vi "Create SBlock (array of pairs).vi"(0 "FPGA Name":string, 5 "Script Path":path, 7 "Common Parameters":T1[](array[typedef]), 9 "Number of repetitions":u16, 11 "error in (no error)":errorcluster) -> (4 "Schedule Block out":refnum<class "Schedule Block.lvclass">, 6 "FPGA Name":string, 15 "error out":errorcluster)   [LabVIEW 2020, in "CIRCUS_uServices.lvlib" / "Run Utilities.lvlib" / "Schedule Block.lvclass"]
uses:
  Schedule Block.lvclass
  Schedule Block.lvclass/Schedule Block.ctl
  TALOS/TALOS_PPL.lvlibp/Interfaces/FPGA Interface/FPGA Interface.lvclass
  TALOS/TALOS_PPL.lvlibp/Support VIs/Global Memory.vi
  TALOS/TALOS_PPL.lvlibp
  Scan SBlock/Parameter name with value - GUI.ctl
  Scan SBlock/Scan SBlock.lvclass
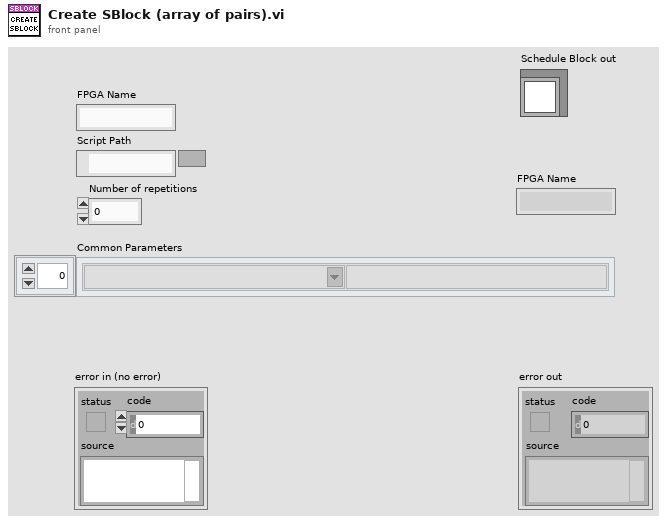
[diagram p1: front panel]
types:
  T1 = typedef "CIRCUS_uServices.lvlib/Run Utilities.lvlib/Scan SBlock.lvclass/Parameter name with value - GUI.ctl" = cluster{"Parameter Name":string, "Parameter Value":string}
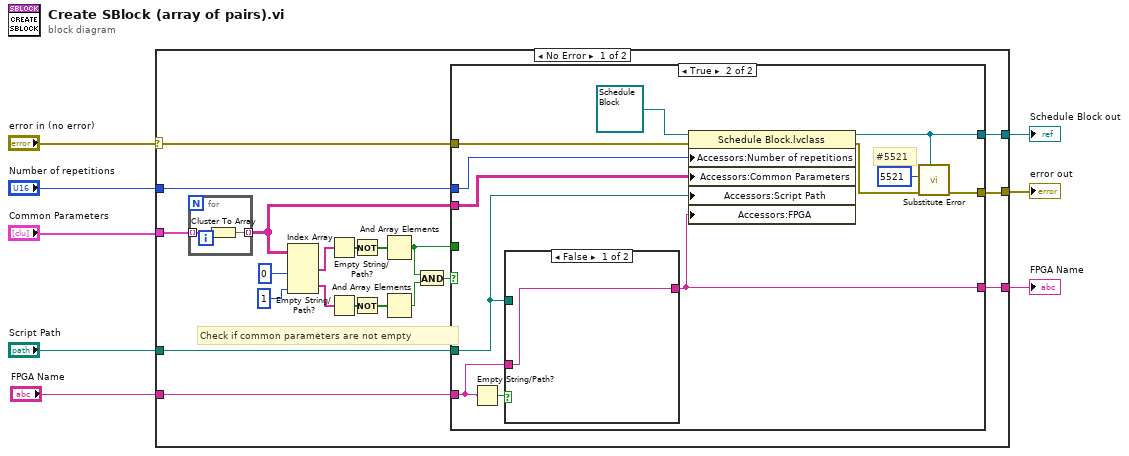
[diagram p0: block diagram]
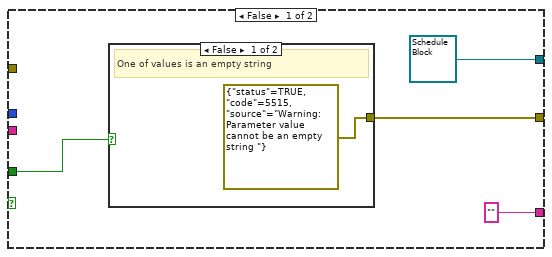
[diagram p2: hidden frame]
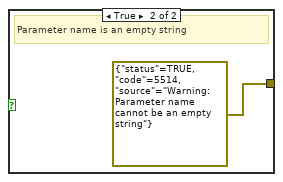
[diagram p3: hidden frame]
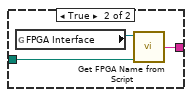
[diagram p4: hidden frame]
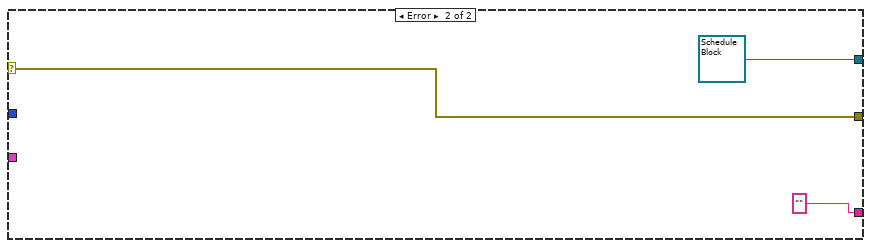
[diagram p5: hidden frame]
diagram:
  n1 = case shown="No Error" "error in (no error)" {
    selector: "error in (no error)" -> [w28 w55]
    tunnel: [w27 w55] -> w7
    tunnel: [w26 refnum<class "Schedule Block.lvclass"> refnum ("Schedule Block in")] -> w6
    tunnel: "Script Path" -> [w25 _]
    tunnel: "Number of repetitions" -> [w24 _]
    tunnel: "Common Parameters" -> [w23 _]
    tunnel: [w10 "" ("Kasli Name")] -> w2
    tunnel: "FPGA Name" -> [w9 _]
    frame No Error {
      # "Check if common parameters are not empty"
      n2 = for {
        tunnel: [w52] -> w18 mode=indexing
        tunnel: w23 -> [w51] mode=indexing
        n3 = Cluster To Array(cluster=w51) -> (array=w52:string[])
      }
      n4 = Index Array(array=w18, index (col) #1=0 ("disabled index (col)"), index (col) #2=1 ("index (col)")) -> (element #1=w20:string[], element #2=w14:string[])  [unwired: 2 in]
      n5 = Empty String/Path?(string/path=w20) -> (empty?=w21:bool[])
      n6 = Empty String/Path?(string/path=w14) -> (empty?=w15:bool[])
      n7 = Not(x=w21) -> (.not. x?=w19:bool[])
      n8 = Not(x=w15) -> (.not. x?=w16:bool[])
      n9 = And Array Elements(Boolean array=w19) -> (logical AND=w11:bool)
      n10 = And Array Elements(Boolean array=w16) -> (logical AND=w13:bool)
      n11 = And(x=w11, y=w13) -> (x .and. y?=w12:bool)
      n12 = case shown="True" w12 {
        tunnel: w28 -> [_ w46]
        tunnel: [w31 w44] -> w27
        tunnel: [refnum<class "Schedule Block.lvclass"> refnum ("Schedule Block in") w42] -> w26
        tunnel: w25 -> [_ w41]
        tunnel: w24 -> [_ w40]
        tunnel: w18 -> [_ w38]
        tunnel: w11 -> [w30 _]
        tunnel: ["" ("Kasli Name") w37] -> w10
        tunnel: w9 -> [_ w35]
        frame False {
          n13 = case shown="False" w30 {
            tunnel: [errorcluster {"status"=TRUE, "code"=5515, "source"="Warning: Parameter value cannot be an empty string "} ("error out") errorcluster {"status"=TRUE, "code"=5514, "source"="Warning: Parameter name cannot be an empty string"} ("error out")] -> w31
            frame False {
              # "One of values is an empty string"
            }
            frame True {
              # "Parameter name is an empty string"
            }
          }
        }
        frame True {
          # "#5521"
          n14 = Empty String/Path?(string/path=w35) -> (empty?=w36:bool)
          n15 = case shown="False" w36 {
            tunnel: w41 -> [_ w50]
            tunnel: [w47 w49] -> w37
            tunnel: w35 -> [w47 _]
            frame False {
            }
            frame True {
              n16 = global read "Global Memory.vi" "FPGA Interface"() -> (w48:refnum<class "FPGA Interface.lvclass">)
              n17 = call-dynamic "Get FPGA Name from Script.vi"("file"=w50, "FPGA Interface"=w48) -> ("FPGA Name"=w49:string)  [unwired: 2 in]
            }
          }
          n18 = property class="Schedule Block.lvclass"(reference=refnum<class "Schedule Block.lvclass"> refnum ("Schedule Block in"), error in=w46, "Accessors:Number of repetitions"=w40, "Accessors:Common Parameters"=w38, "Accessors:Script Path"=w41, "Accessors:FPGA"=w37) -> (reference out=w42:refnum<class "Schedule Block.lvclass">, error out=w45:errorcluster)
          n19 = call "Substitute Error.vi"("LabVIEW Object"=w42, "error in (no error)"=w45, "Error Code"=5521) -> ("error out"=w44:errorcluster)  [unwired: 8 in]
        }
      }
    }
    frame Error {
    }
  }
  "error out" <- w7
  "Schedule Block out" <- w6
  "FPGA Name" <- w2
